vi "IMIC_SetZPosAbs.vi"(2 "zpos":dbl format="%^#_6g", 3 "index":i32, 4 "handle":u64) -> (0 "handle out":u64, 1 "output param":T1(ring))   [LabVIEW 2011]
uses:
  tillimic64.dll
panel:
  out "indexout":i32
  # "running untill reached"
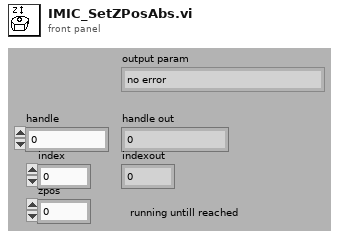
[diagram p1: front panel]
types:
  T1 = enum16{"no error", "missing axis", "missing Z axis", "missing Filter", "iMic not initialized", "no property", "wrong handle", "protocol not finished", "user parameter to long (>32 bits)", "no user parameter handle", "failed to open comport", "failed to initialize"}
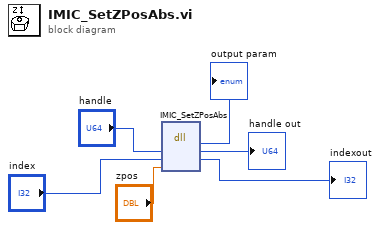
[diagram p0: block diagram]
diagram:
  n1 = dll-call lib="C:/Program Files/colibri/Drivers/TILLPhotonics/tillimic*.*" fn="IMIC_SetZPosAbs"("handle"="handle", "index"="index", "zpos"="zpos") -> ("return type"=→"output param":i32, "handle"=→"handle out":u64, "index"=→"indexout":i32)  [unwired: 4 in, 2 out]
